vi "Initialize Owner Attribute.vi"(9 "Shared Key":string, 10 "Owner GUID":string, 11 "Owner Name":string) -> (3 "Attribute.Owner":refnum<class "Attribute.Owner.lvclass">)   [LabVIEW 2021, in "smo.lvlib" / "Attribute.Owner.lvclass"]
uses:
  Attribute.Owner.lvclass
  C:/Repositories/SMO/src/Support/Attribute/Attribute.lvclass
  Packet -- Cluster.ctl
  Definitions/def.SMO/Scope -- Enum.ctl
  Attribute.Owner.lvclass/Attribute.Owner.ctl
  Attribute/Attribute.lvclass/Attribute.ctl
  Definitions/def.SMO/def.SMO.lvclass
  Attribute/Attribute.lvclass
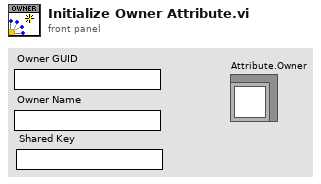
[diagram p1: front panel]
types:
  T1 = typedef "smo.lvlib/def.SMO.lvclass/Scope -- Enum.ctl" = enum16{"Public", "Protected", "Private"}
  T2 = typedef "smo.lvlib/Attribute.Owner.lvclass/Packet -- Cluster.ctl" = cluster{"Message":string, "Payload":variant, "Source GUID":string}
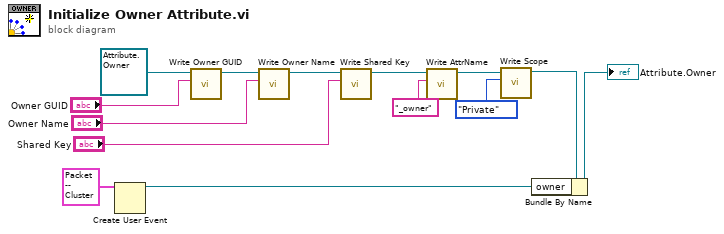
[diagram p0: block diagram]
diagram:
  n1 = Create User Event(user event datatype=T2 {"Message"="", "Payload"=variant, "Source GUID"=""} ("Packet")) -> (user event=w7:refnum<user-event>)  [unwired: 1 in, 1 out]
  n2 = call "Write Owner GUID.vi"("Owner GUID"="Owner GUID", "Attribute.Owner in"=refnum<class "Attribute.Owner.lvclass"> refnum) -> ("Attribute.Owner out"=w13:refnum<class "Attribute.Owner.lvclass">)  [unwired: 8 in, 1 out]
  n3 = call "Write Owner Name.vi"("Owner Name"="Owner Name", "Attribute.Owner in"=w13) -> ("Attribute.Owner out"=w12:refnum<class "Attribute.Owner.lvclass">)  [unwired: 8 in, 1 out]
  n4 = call "Write Shared Key.vi"("Shared Key"="Shared Key", "Attribute.Owner in"=w12) -> ("Attribute.Owner out"=w5:refnum<class "Attribute.Owner.lvclass">)  [unwired: 8 in, 1 out]
  n5 = call "Write AttrName.vi"("Attribute Name"="_owner" ("Name"), "Attribute in"=w5) -> ("Attribute out"=w4:refnum<class "Attribute.Owner.lvclass">)  [unwired: 9 in]
  n6 = call "Write Scope.vi"("Scope"=Scope_--_Enum."Private", "Attribute in"=w4) -> ("Attribute out"=w3:refnum<class "Attribute.Owner.lvclass">)  [unwired: 9 in]
  n7 = Bundle By Name(cluster=w3, "owner"=w7) -> (→"Attribute.Owner":refnum<class "Attribute.Owner.lvclass">)
